vi "Restart Cameras.vi"() -> (0 "Error Out":errorcluster)   [LabVIEW 2015]
panel:
  out "cmd string":string
  in  "Batch filename":string="Restart Cameras (runAs Administrator)"
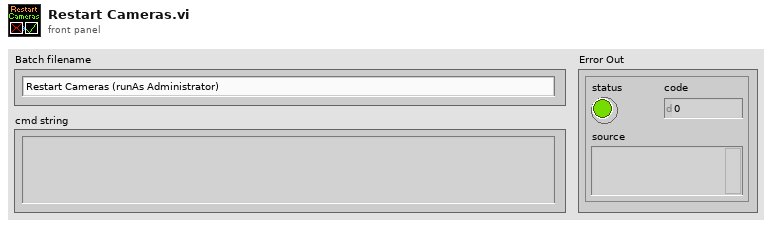
[diagram p1: front panel]
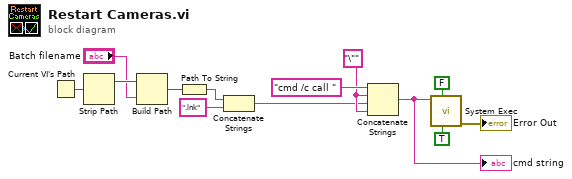
[diagram p0: block diagram]
diagram:
  w6 = "\"" ("string")
  n1 = Current VI's Path() -> (path=w10:path)
  n2 = Strip Path(path=w10) -> (stripped path=w9:path)  [unwired: 1 out]
  n3 = Build Path(base path=w9, name or relative path="Batch filename") -> (appended path=w7:path)
  n4 = Path To String(path=w7) -> (string=w4:string)
  n5 = Concatenate Strings(w4, ".lnk" ("string")) -> (w2:string)
  n6 = Concatenate Strings("cmd /c call ", w6, w2, w6) -> (w5:string)
  "cmd string" <- w5
  n7 = call <vilib>:"System Exec.vi"("run minimized? (F)"=TRUE, "wait until completion? (T)"=FALSE, "command line"=w5) -> ("error out"=→"Error Out":errorcluster)  [unwired: 5 in, 3 out]
